vi "Find All Zeros of f(x).vi"   [LabVIEW 2012, in "NI_Gmath.lvlib"]
doc: "Determines all zeros of a 1D function in a given interval. You must manually select the polymorphic instance to use."
uses:
  NI_Gmath.lvlib
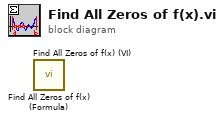
[diagram p0: block diagram]
diagram:
  n1 = call "Find All Zeros of f(x) (Formula).vi"() -> ()  [unwired: 8 in, 4 out]
  n2 = call "Find All Zeros of f(x) (VI).vi"() -> ()  [unwired: 8 in, 4 out]
